vi "JoystickDeadZone.vi"(9 "scale":dbl, 10 "dead zone":dbl, 11 "input variable":dbl(slide) scale=-2.0..2.0) -> (2 "output variable":dbl)   [LabVIEW 2015]
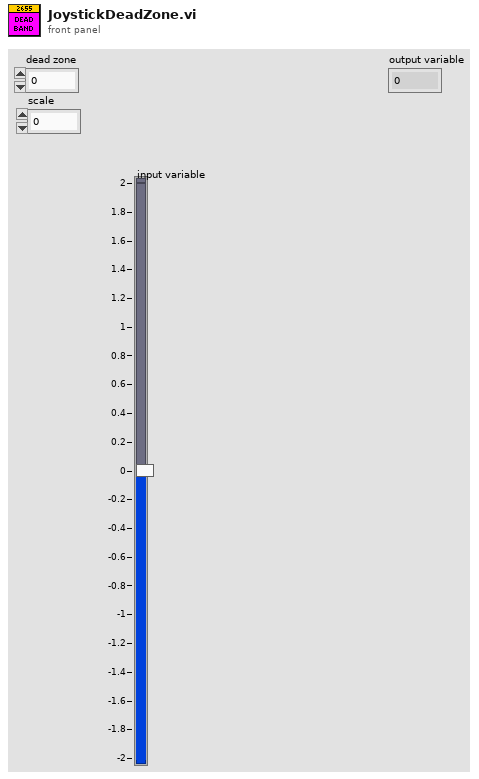
[diagram p1: front panel]
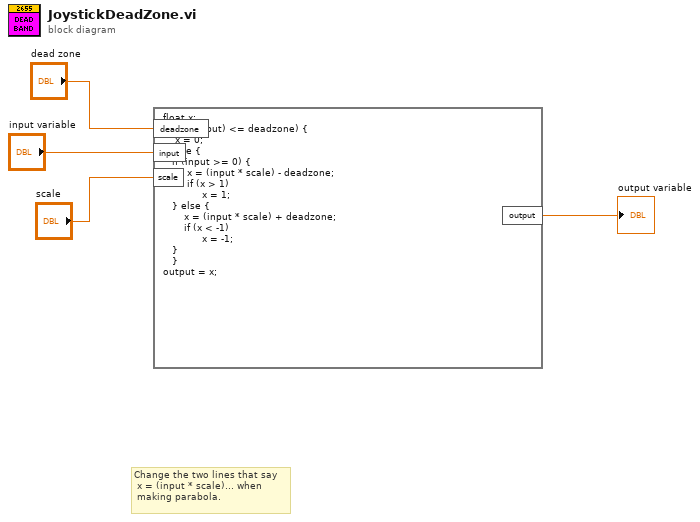
[diagram p0: block diagram]
diagram:
  # "Change the two lines that say\n x = (input * scale)... when\n making parabola."
  n1 = formula code="float x;\nif (abs(input) <= deadzone) {\n    x = 0;\n} else {\n   if (input >= 0) {\n        x = (input * scale) - deadzone;\n        if (x > 1)\n             x = 1;\n   } else {\n       x = (input * scale) + deadzone;\n       if (x < -1)\n             x = -1;\n   }\n   }\noutput = x;"("deadzone"="dead zone", "scale"="scale", "input"="input variable") -> ("output"=→"output variable":dbl)
